vi "Autonomous Independent.vi"   [LabVIEW 2019]
doc: "This VI is called when autonomous begins, and will automatically be terminated when autonomous ends. You can carry out timed or sensor driven robot movement independently without needing to return to the caller."
uses:
  <vilib>/Rock Robotics/Network Tables/NT Read Number.vi
  <vilib>/Rock Robotics/Network Tables/NT Read String.vi
  Robot Global Data.vi
panel:
  # "Be sure to right-click and choose Data Operations>>Make Current Value default if you want to save the array values with the VI"
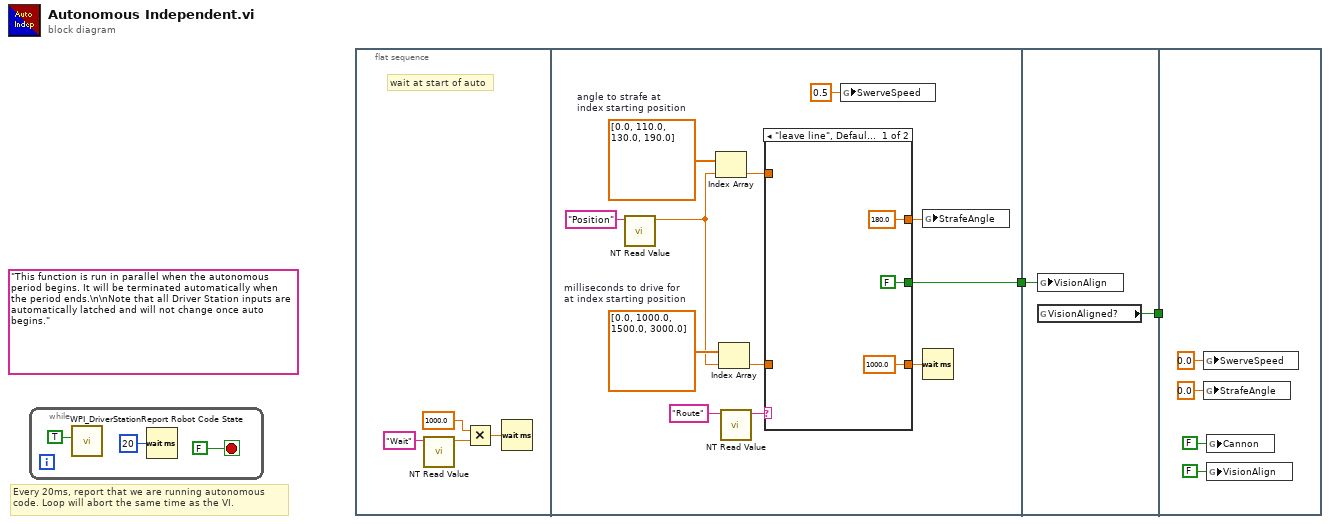
[diagram p0: block diagram]
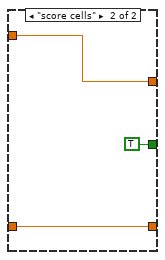
[diagram p2: hidden frame]
diagram:
  (unwired) "This function is run in parallel when the autonomous period begins. It will be terminated automatically when the period ends.\n\nNote that all Driver Station inputs are automatically latched and will not change once auto begins."
  # "Every 20ms, report that we are running autonomous\ncode. Loop will abort the same time as the VI."
  n1 = while {
    stop <- FALSE stop-if-true
    n2 = call <vilib>:"WPI_DriverStationReport Robot Code State.vi"("Autonomous"=TRUE) -> ()  [unwired: 10 in, 1 out]
    n3 = Wait (ms)(milliseconds to wait=u32 20) -> ()  [unwired: 1 out]
  }
  n4 = flat-sequence {
    tunnel: [w10] -> w2
    tunnel: w2 -> [w29]
    tunnel: [w28] -> w1
    tunnel: w1 -> [_]
    frame #0 {
      # "wait at start of auto"
      n5 = call-poly <vilib>:"NT Read Value.vi"("Name"="Wait") -> ("Numeric"=w8:dbl)  [unwired: 9 in, 1 out]
      n6 = Multiply(x=1000.0, y=w8) -> (x*y=w7:dbl)
      n7 = Wait (ms)(milliseconds to wait=w7) -> ()  [unwired: 1 out]
    }
    frame #1 {
      w13 = dbl[] [0.0, 1000.0, 1500.0, 3000.0]  # milliseconds to drive for at index starting position
      w19 = dbl[] [0.0, 110.0, 130.0, 190.0]  # angle to strafe at index starting position
      n8 = call-poly <vilib>:"NT Read Value.vi"("Name"="Position") -> ("Numeric"=w12:dbl)  [unwired: 9 in, 1 out]
      n9 = Index Array(array=w19, index=w12) -> (element=w18:dbl)
      n10 = Index Array(array=w13, index=w12) -> (element=w11:dbl)
      n11 = call-poly <vilib>:"NT Read Value.vi"("Name"="Route") -> ("String"=w17:string)  [unwired: 9 in, 1 out]
      n12 = case shown="\"leave line\", Default" w17 {
        tunnel: [180.0 w27] -> w16
        tunnel: w18 -> [_ w27]
        tunnel: [1000.0 w26] -> w14
        tunnel: w11 -> [_ w26]
        tunnel: [FALSE TRUE] -> w10
        frame "leave line", Default {
        }
        frame "score cells" {
        }
      }
      n13 = global write "Robot Global Data.vi" "SwerveSpeed"(0.5 ("SwerveSpeed")) -> ()
      n14 = global write "Robot Global Data.vi" "StrafeAngle"(w16) -> ()
      n15 = Wait (ms)(milliseconds to wait=w14) -> ()  [unwired: 1 out]
    }
    frame #2 {
      n16 = global write "Robot Global Data.vi" "VisionAlign"(w29) -> ()
      n17 = global read "Robot Global Data.vi" "VisionAligned?"() -> (w28:bool)
    }
    frame #3 {
      n18 = global write "Robot Global Data.vi" "SwerveSpeed"(0.0 ("SwerveSpeed")) -> ()
      n19 = global write "Robot Global Data.vi" "StrafeAngle"(0.0 ("StrafeAngle")) -> ()
      n20 = global write "Robot Global Data.vi" "Cannon"(FALSE ("Cannon")) -> ()
      n21 = global write "Robot Global Data.vi" "VisionAlign"(FALSE ("VisionAlign")) -> ()
    }
  }
